vi "Generate Unique Header.vi"(8 "error in (no error)":errorcluster, 11 "CRDS Data in":refnum<class "CRDS Data.lvclass">) -> (0 "error out":errorcluster, 2 "Header":string[](array[string]), 3 "CRDS Data out":refnum<class "CRDS Data.lvclass">)   [LabVIEW 2014, in "CRDS Data.lvclass"]
uses:
  CRDS Data.lvclass
  CRDS Data.lvclass/CRDS Data.ctl
  Cell/CRDS Cell Data.lvclass
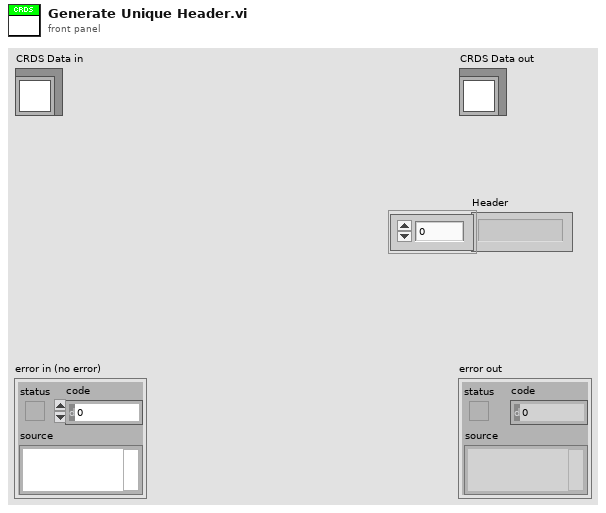
[diagram p1: front panel]
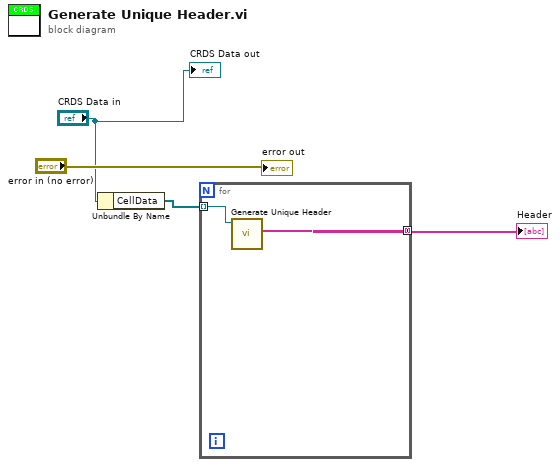
[diagram p0: block diagram]
diagram:
  n1 = Unbundle By Name("CRDS Data in") -> ("CellData"=w4:refnum<class "CRDS Cell Data.lvclass">[])
  n2 = for {
    tunnel: w4 -> [w6] mode=indexing
    tunnel: [w5] -> w3 mode=concatenating
    n3 = call-dynamic "Generate Unique Header.vi"("CRDS Cell Data in"=w6) -> ("Header"=w5:string[])  [unwired: 8 in, 2 out]
  }
  "Header" <- w3
  "error out" <- "error in (no error)"
  "CRDS Data out" <- "CRDS Data in"
